vi "Read Attributes.vi"(11 "Start Microgrid Msg":refnum<class "Start Microgrid Msg.lvclass">) -> (2 "Payload":cluster{"Data":variant})   [LabVIEW 2018, in "Remote Operation Abstract.lvlib" / "Start Microgrid Msg.lvclass"]
uses:
  Start Microgrid Msg.lvclass
  Start Microgrid Msg.lvclass/Start Microgrid Msg.ctl
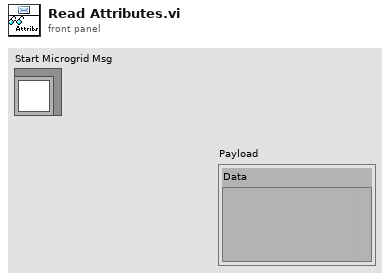
[diagram p1: front panel]
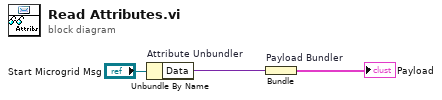
[diagram p0: block diagram]
diagram:
  n1 = Unbundle By Name "Attribute Unbundler"("Start Microgrid Msg") -> ("Data"=w1:variant)
  n2 = Bundle "Payload Bundler"("Data"=w1) -> (→"Payload":cluster{"Data":variant})  [unwired: 1 in]
